vi "Construct message class.vi"(8 "error in (no error)":errorcluster, 11 "object in":refnum<class "Message Class.lvclass">) -> (0 "error out":errorcluster, 3 "object out":refnum<class "Message Class.lvclass">)   [LabVIEW 2018, in "ClientMessaging.lvlib" / "Message Class.lvclass"]
doc: "Construct a message class or sub class from the header"
uses:
  Message Class.lvclass
  Message Class.lvclass/Message Class.ctl
  <vilib>/regexp/Match Regular Expression.xnode
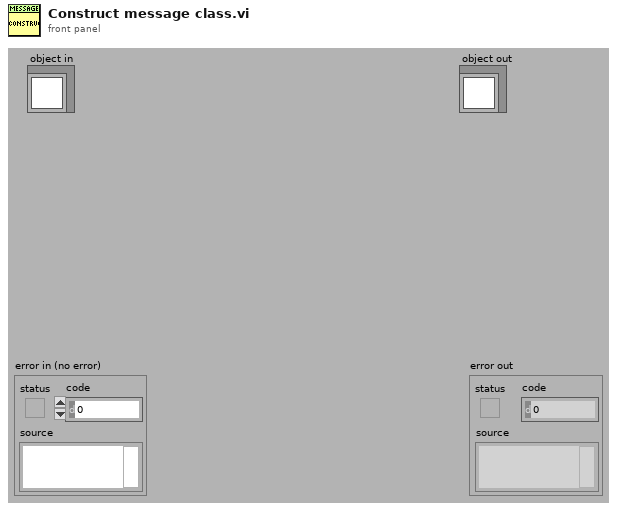
[diagram p1: front panel]
types:
  T1 = typedef "ClientMessaging.lvlib/Message Class.lvclass/header_dict.ctl" = cluster{"msg_id":string, "username":string, "session":string, "date":timestamp, "msg_type":string, "version":string}
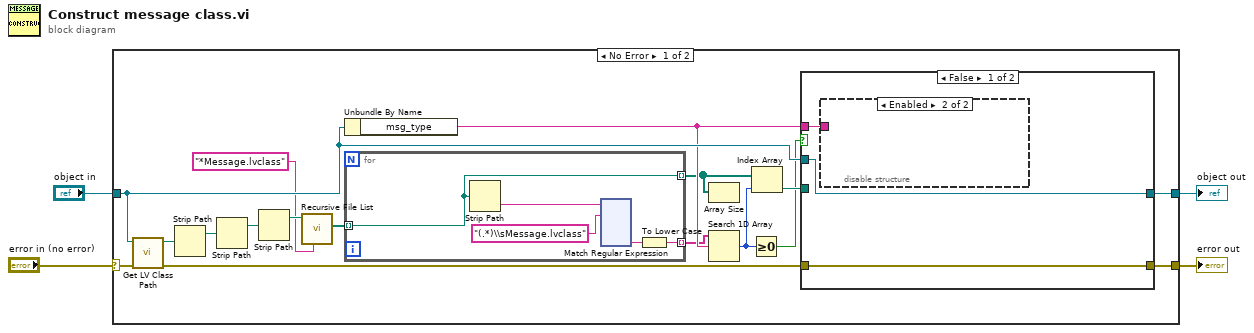
[diagram p0: block diagram]
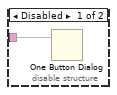
[diagram p2: hidden frame]
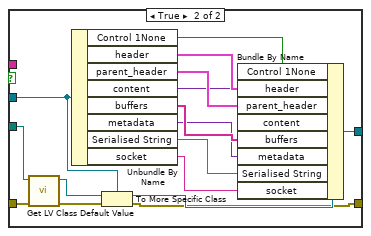
[diagram p3: hidden frame]
diagram:
  n1 = case shown="No Error" "error in (no error)" {
    selector: "error in (no error)" -> [w19 w164]
    tunnel: [w18 w164] -> w3
    tunnel: [w20 w163] -> w1
    tunnel: "object in" -> [w21 w163]
    frame No Error {
      n2 = call <vilib>:"Get LV Class Path.vi"("error in (no error)"=w19, "object"=w21) -> ("error out"=w13:errorcluster, "class path"=w11:path)  [unwired: 8 in]
      n3 = Strip Path(path=w11) -> (stripped path=w10:path)  [unwired: 1 out]
      n4 = Strip Path(path=w10) -> (stripped path=w6:path)  [unwired: 1 out]
      n5 = Strip Path(path=w6) -> (stripped path=w9:path)  [unwired: 1 out]
      n6 = call <vilib>:"Recursive File List.vi"("pattern"="*Message.lvclass", "Folder Path"=w9) -> ("All Files in Dir"=w7:path[])  [unwired: 5 in, 4 out]
      n7 = Unbundle By Name(w21) -> ("msg_type"=w17:string)
      n8 = for {
        tunnel: w7 -> [w23] mode=indexing
        tunnel: [w22] -> w12 mode=indexing
        tunnel: [w23] -> w5 mode=indexing
        n9 = Strip Path(path=w23) -> (name=w26:string)  [unwired: 1 out]
        n10 = xnode "Match Regular Expression"("input string"=w26, "regular expression"="(.*)\\sMessage.lvclass") -> ("submatch 1"=w24:string)  [unwired: 4 in, 5 out]
        n11 = To Lower Case(string=w24) -> (all lower case string=w22:string)
      }
      n12 = Array Size(array=w5) -> ()  [unwired: 1 out]
      n13 = Search 1D Array(1D array=w12, element=w17) -> (index of element=w16:i32)  [unwired: 1 in]
      n14 = Greater Or Equal To 0?(x=w16) -> (x >= 0?=w14:bool)
      n15 = Index Array(array=w5, index=w16) -> (element=w15:path)
      n16 = case shown="False" w14 {
        tunnel: w13 -> [w144 w162]
        tunnel: w15 -> [_ w161]
        tunnel: w21 -> [w145 w156]
        tunnel: [w145 w155] -> w20
        tunnel: [w144 w157] -> w18
        tunnel: w17 -> [w143 _]
        frame False {
          n17 = disable-structure shown="Enabled" {
            disable-tunnel: w143 -> [w146 _]
            frame Disabled {
              n18 = One Button Dialog(message=w146) -> ()  [unwired: 1 in, 1 out]
            }
            frame Enabled {
            }
          }
        }
        frame True {
          n19 = call <vilib>:"Get LV Class Default Value.vi"("error in (no error)"=w162, "class path"=w161) -> ("error out"=w159:errorcluster, "object"=w160:refnum<class>)  [unwired: 8 in]
          n20 = Unbundle By Name(w156) -> ("Control 1None"=w154:bool, "header"=w153:T1, "parent_header"=w152:T1, "content"=w151:variant, "buffers"=w150:string[], "metadata"=w149:variant, "Serialised String"=w148:string, "socket"=w147:string)
          n21 = To More Specific Class(target class=w156, reference=w160, error in=w159) -> (specific class reference=w158:refnum<class "Message Class.lvclass">, error out=w157:errorcluster)
          n22 = Bundle By Name(cluster=w158, "Control 1None"=w154, "header"=w153, "parent_header"=w152, "content"=w151, "buffers"=w150, "metadata"=w149, "Serialised String"=w148, "socket"=w147) -> (w155:refnum<class "Message Class.lvclass">)
        }
      }
    }
    frame Error {
    }
  }
  "error out" <- w3
  "object out" <- w1
